vi "Clear_Lines-RINSE.vi"   [LabVIEW 2019]
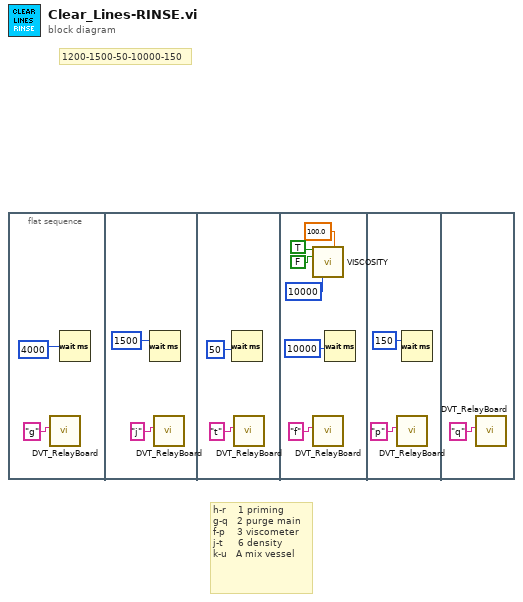
[diagram p0: block diagram]
diagram:
  # "1200-1500-50-10000-150"
  # "h-r    1 priming\ng-q   2 purge main\nf-p    3 viscometer\nj-t     6 density\nk-u   A mix vessel"
  n1 = flat-sequence {
    frame #0 {
      n2 = call "DVT_RelayBoard.vi"("write buffer"="g") -> ()  [unwired: 3 in, 3 out]
      n3 = Wait (ms)(milliseconds to wait=u32 4000) -> ()  [unwired: 1 out]
    }
    frame #1 {
      n4 = Wait (ms)(milliseconds to wait=u32 1500) -> ()  [unwired: 1 out]
      n5 = call "DVT_RelayBoard.vi"("write buffer"="j") -> ()  [unwired: 3 in, 3 out]
    }
    frame #2 {
      n6 = Wait (ms)(milliseconds to wait=u32 50) -> ()  [unwired: 1 out]
      n7 = call "DVT_RelayBoard.vi"("write buffer"="t") -> ()  [unwired: 3 in, 3 out]
    }
    frame #3 {
      n8 = call "VISCOSITY.vi"("SPIN (F)"=TRUE ("SPIN"), "Startup RPM"=100.0, "LogData? (T)"=FALSE ("LogData?"), "stabilization (ms)"=u32 10000) -> ()  [unwired: 5 in, 7 out]
      n9 = call "DVT_RelayBoard.vi"("write buffer"="f") -> ()  [unwired: 3 in, 3 out]
      n10 = Wait (ms)(milliseconds to wait=u32 10000) -> ()  [unwired: 1 out]
    }
    frame #4 {
      n11 = call "DVT_RelayBoard.vi"("write buffer"="p") -> ()  [unwired: 3 in, 3 out]
      n12 = Wait (ms)(milliseconds to wait=u32 150) -> ()  [unwired: 1 out]
    }
    frame #5 {
      n13 = call "DVT_RelayBoard.vi"("write buffer"="q") -> ()  [unwired: 3 in, 3 out]
    }
  }
